vi "Set Channel Group Channel Names.vi"(8 "error in (no error)":errorcluster, 10 "names":string[](array[string]), 11 "channel group in":T1 format="%.0x") -> (0 "error out":errorcluster, 3 "channel group out":T1 format="%.0x")   [LabVIEW 2027, in "Embedded Data Logger Scripting.lvlib"]
uses:
  Embedded Data Logger Scripting.lvlib
  <vilib>/NI VeriStand/Custom Device API/Custom Device Item Ref.ctl
  <vilib>/NI VeriStand/Custom Device API/Set Item Property (String Array).vi
  <vilib>/NI VeriStand/Custom Device API/Custom Device API.lvlib
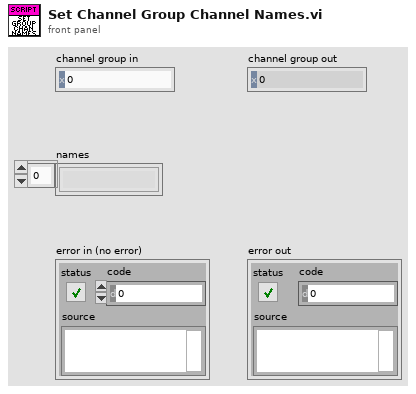
[diagram p1: front panel]
types:
  T1 = typedef "Custom Device API.lvlib/Custom Device Item Ref.ctl" = u64
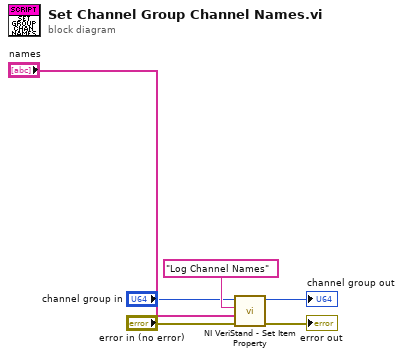
[diagram p0: block diagram]
diagram:
  n1 = call-poly <vilib>:"NI VeriStand - Set Item Property.vi"("error in (no error)"="error in (no error)", "Value"="names", "Property Name"="Log Channel Names", "Item Ref in"="channel group in") -> ("error out"=→"error out":errorcluster, "Item Ref out"=→"channel group out":T1)  [unwired: 5 in, 1 out]
